vi "Launcher.vi"() -> ()   [LabVIEW 2023]
uses:
  Table/Table/Table.lvclass
  C:/Program Files (x86)/National Instruments/LabVIEW 2023/vi.lib/ActorFramework/Actor/Actor.lvclass
  Table/Table/Table.lvclass/Table.ctl
  <vilib>/ActorFramework/Actor/Actor.lvclass
panel:
  in  "# Philosophers":i32=5 min=5 max=500 step=1
  # "Overview:  https://en.wikipedia.org/wiki/Dining_philosophers_problem\n\nRequirements:  LabVIEW 2023 Q1\n\nInstructions:  Run the VI."
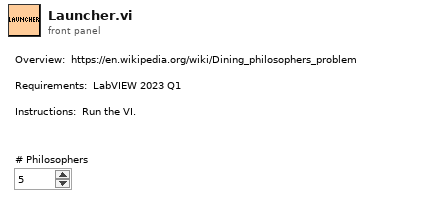
[diagram p1: front panel]
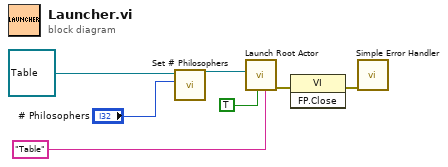
[diagram p0: block diagram]
diagram:
  n1 = call "Set # Philosophers.vi"("# Philosophers"="# Philosophers", "Table in"=refnum<class "Table.lvclass"> refnum ("Table.lvlib:Table.lvclass")) -> ("Table out"=w3:refnum<class "Table.lvclass">)  [unwired: 8 in, 1 out]
  n2 = call <vilib>:"Launch Root Actor.vi"("Debug Alias"="Table", "Open Actor Core front panel? (F)"=TRUE, "Actor"=w3) -> ("error out"=w6:errorcluster)  [unwired: 7 in, 1 out]
  n3 = invoke class="VI" method="FP.Close"(error in=w6) -> (error out=w7:errorcluster)  [unwired: 2 in, 2 out]
  n4 = call <vilib>:"Simple Error Handler.vi"("error in (no error)"=w7) -> ()  [unwired: 4 in, 5 out]
